vi "Functional Imaging-Generate viewer menu.vi"() -> (0 "error out":errorcluster, 3 "Functional Viewer Menu":refnum<k9>)   [LabVIEW 2020]
uses:
  Global variables/gl_Functional Imaging-Global variables.vi
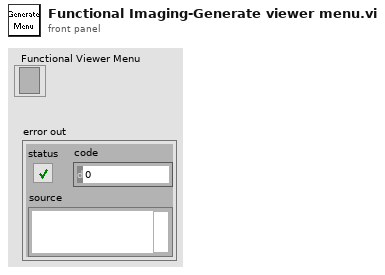
[diagram p1: front panel]
types:
  T1 = typedef "Functional Imging UI Refs.ctl" = cluster{"Menu ref":refnum<k9>, "Image control":refnum<vi>, "VI ref":refnum<vi>, "XGrapher":refnum<vi>, "Smoothing":refnum<vi>, "POI Averaging":refnum<vi>, "Normalize":refnum<vi>, "POI data points in each trial":refnum<vi>, "Channel":refnum<vi>, "Experiment data folder path":refnum<vi>, "[ROI vis]":refnum<vi>, "[Groups] visbl":T2, "Group Name":refnum<vi>, "POI index":refnum<vi>, "Trial No.":refnum<vi>, "Intensity Zoom":refnum<vi>, "Trial Cursor Enabled":refnum<vi>, "Number of Trials (ind 1)":refnum<vi>, "Number of Trials (ind 2)":refnum<vi>, "MiniScans Available":refnum<vi>, "POI Available":refnum<vi>, "Defer graph updates":refnum<vi>, "Waveform selector":refnum<vi>, "#of selected POI":refnum<vi>, "#of selected MiniScans":refnum<vi>, "#of selected groups":refnum<vi>, "Max Z-Projection":refnum<vi>, "Z-Plane Selector":refnum<vi>, "Index of miniscan point to visualise":refnum<vi>, "ROI vis. mode":refnum<vi>, "Total # of points":refnum<vi>, "Index of group clicked on":refnum<vi>, "Pane 1":refnum<vi>, "Pane 2":refnum<vi>, "Pane 3":refnum<vi>, "Pane 4":refnum<vi>, "Pane 5":refnum<vi>, "Pane 6":refnum<vi>, "Deselect all ROI":refnum<vi>, "Deselect all groups":refnum<vi>}
  T2 = typedef "Groups array referecne.ctl" = refnum<vi>
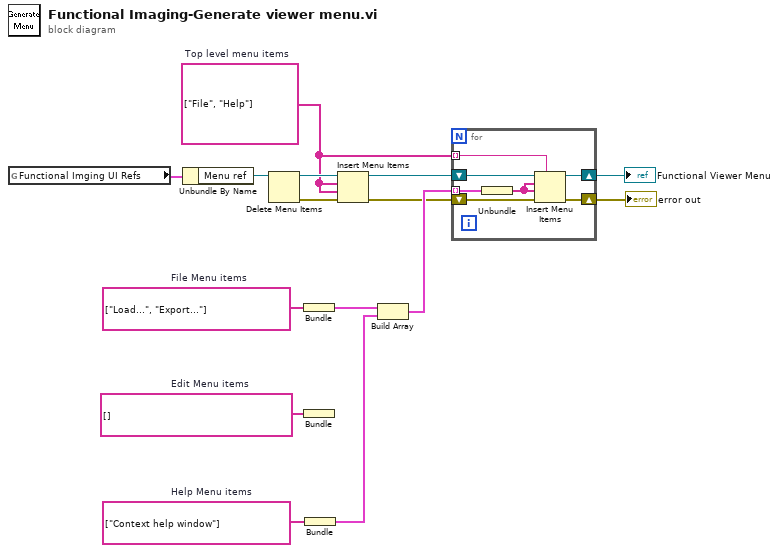
[diagram p0: block diagram]
diagram:
  w8 = string[] ["Context help window"]  # Help Menu items
  w9 = string[] []  # Edit Menu items
  w11 = string[] ["Load...", "Export..."]  # File Menu items
  w12 = string[] ["File", "Help"]  # Top level menu items
  n1 = global read "gl_Functional Imaging-Global variables.vi" "Functional Imging UI Refs"() -> (w2:T1)
  n2 = Unbundle By Name(w2) -> ("Menu ref"=w1:refnum<k9>)
  n3 = Delete Menu Items(9:w1) -> (0:w15:errorcluster, 3:w14:refnum<k9>)  [unwired: 3 in]
  n4 = Bundle("File Menu items"=w11) -> (w10:cluster{"File Menu items":string[]})  [unwired: 1 in]
  n5 = Bundle("Edit Menu items"=w9) -> ()  [unwired: 1 in, 1 out]
  n6 = Bundle("Help Menu items"=w8) -> (w3:cluster{"Help Menu items":string[]})  [unwired: 1 in]
  n7 = Insert Menu Items(6:w15, 7:w12, 8:w12, 9:w14) -> (0:w4:errorcluster, 3:w13:refnum<k9>)  [unwired: 2 in, 1 out]
  n8 = Build Array(w10, w3) -> (w7:cluster{"Help Menu items":string[]}[])
  n9 = for {
    shift-right: [w21] -> w6
    shift-left: w13 -> [w22]
    tunnel: w12 -> [w20] mode=indexing
    tunnel: w7 -> [w19] mode=indexing
    shift-right: [w17] -> w5
    shift-left: w4 -> [w16]
    n10 = Unbundle(w19) -> ("Help Menu items"=w18:string[])
    n11 = Insert Menu Items(5:w20, 6:w16, 7:w18, 8:w18, 9:w22) -> (0:w17:errorcluster, 3:w21:refnum<k9>)  [unwired: 1 in, 1 out]
  }
  "error out" <- w5
  "Functional Viewer Menu" <- w6
